vi "Convert64PinPGAToPattern.vi"(11 "64-Pin PGA":T3) -> (3 "Pattern":T1)   [LabVIEW 2012, in "Virtual-PGA.lvlib"]
uses:
  Virtual-PGA.lvlib
  Public/Controls/64PinPGAPattern.ctl
  Public/Controls/64PinPGAPads1-16.ctl
  Public/Controls/64PinPGAPad1-16.ctl
  Public/Controls/64PinPGAPads17-32.ctl
  Public/Controls/64PinPGAPad17-32.ctl
  Public/Controls/64PinPGAPads33-48.ctl
  Public/Controls/64PinPGAPad33-48.ctl
  Public/Controls/64PinPGAPads49-64.ctl
  Public/Controls/64PinPGAPad49-64.ctl
  Public/Controls/Pattern.ctl
  Public/Controls/Input.ctl
panel:
  # "Name:"
  # "Inputs:"
  # "Description:"
  # "Y4:"
  # "Y3:"
  # "Y2:"
  # "Y1:"
  # "49"
  # "50"
  # "51"
  # "52"
  # "53"
  # "54"
  # "55"
  # "56"
  # "57"
  # "58"
  # "59"
  # "60"
  # "61"
  # "62"
  # "63"
  # "64"
  # "1"
  # "2"
  # "3"
  # "4"
  # "5"
  # "6"
  # "7"
  # "8"
  # "9"
  # "10"
  # "11"
  # "12"
  # "13"
  # "14"
  # "15"
  # "16"
  # "32"
  # "31"
  # "30"
  # "29"
  # "28"
  # "27"
  # "26"
  # "25"
  # "24"
  # "23"
  # "22"
  # "21"
  # "20"
  # "19"
  # "18"
  # "17"
  # "48"
  # "47"
  # "46"
  # "45"
  # "44"
  # "43"
  # "42"
  # "41"
  # "40"
  # "39"
  # "38"
  # "37"
  # "36"
  # "35"
  # "34"
  # "33"
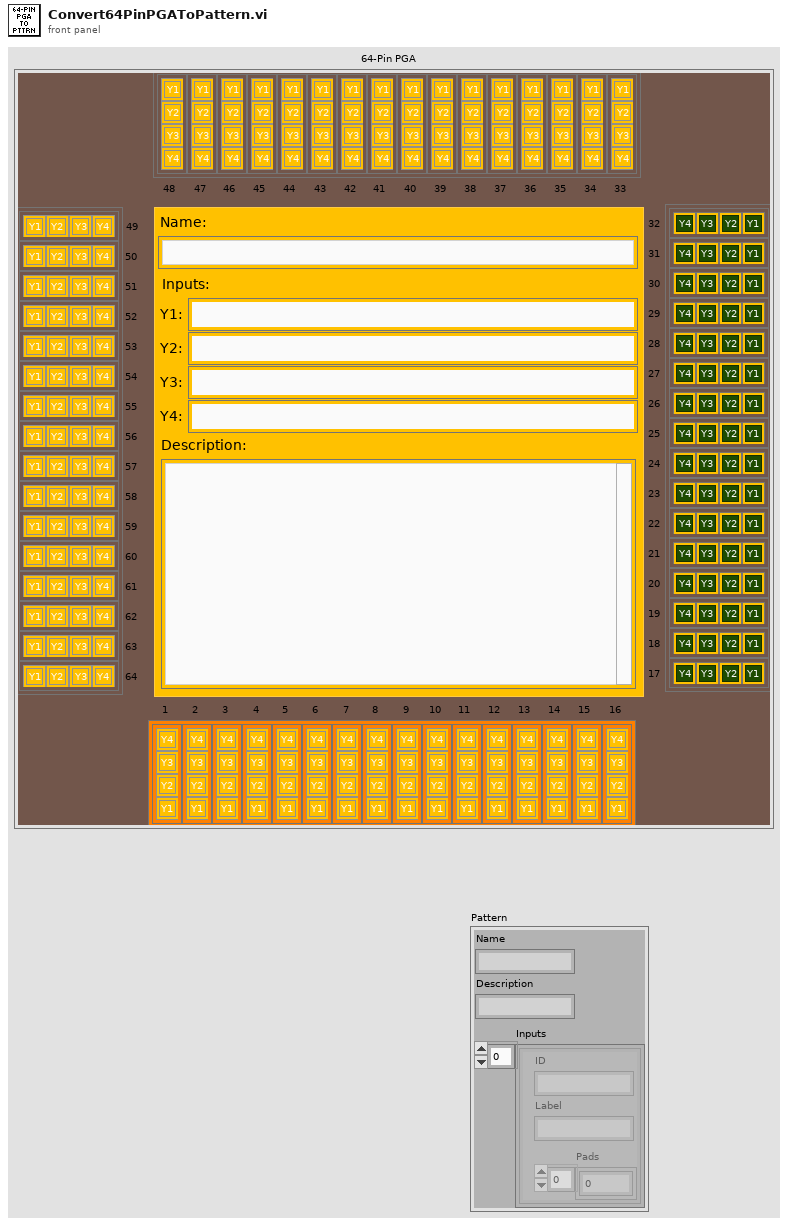
[diagram p1: front panel]
types:
  T1 = typedef "Virtual-PGA.lvlib/Pattern.ctl" = cluster{"Name":string, "Description":string, "Inputs":T2[]}
  T2 = typedef "Virtual-PGA.lvlib/Input.ctl" = cluster{"ID":string, "Label":string, "Pads":u32[]}
  T3 = typedef "Virtual-PGA.lvlib/64PinPGAPattern.ctl" = cluster{"Name":string, "Description":string, "Y1 Label":string, "Y2 Label":string, "Y3 Label":string, "Y4 Label":string, "Pads 1-16":T4, "Pads 17-32":T6, "Pads 33-48":T8, "Pads 49-64":T10}
  T4 = typedef "Virtual-PGA.lvlib/64PinPGAPads1-16.ctl" = T5[]
  T5 = typedef "Virtual-PGA.lvlib/64PinPGAPad1-16.ctl" = cluster{"Y1":bool, "Y2":bool, "Y3":bool, "Y4":bool}
  T6 = typedef "Virtual-PGA.lvlib/64PinPGAPads17-32.ctl" = T7[]
  T7 = typedef "Virtual-PGA.lvlib/64PinPGAPad17-32.ctl" = cluster{"Y1":bool, "Y2":bool, "Y3":bool, "Y4":bool}
  T8 = typedef "Virtual-PGA.lvlib/64PinPGAPads33-48.ctl" = T9[]
  T9 = typedef "Virtual-PGA.lvlib/64PinPGAPad33-48.ctl" = cluster{"Y1":bool, "Y2":bool, "Y3":bool, "Y4":bool}
  T10 = typedef "Virtual-PGA.lvlib/64PinPGAPads49-64.ctl" = T11[]
  T11 = typedef "Virtual-PGA.lvlib/64PinPGAPad49-64.ctl" = cluster{"Y1":bool, "Y2":bool, "Y3":bool, "Y4":bool}
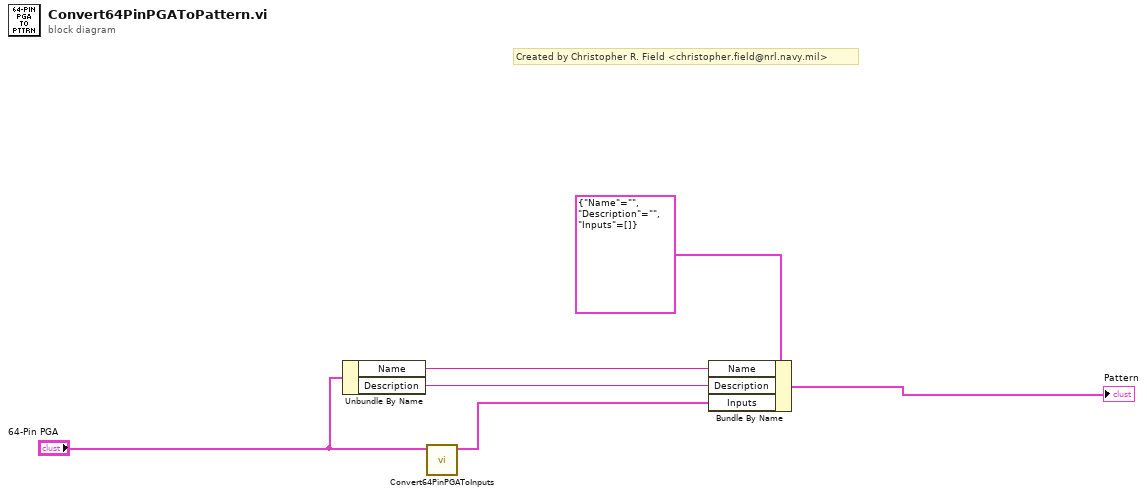
[diagram p0: block diagram]
diagram:
  # "Created by Christopher R. Field <christopher.field@nrl.navy.mil>"
  n1 = Unbundle By Name("64-Pin PGA") -> ("Name"=w3:string, "Description"=w2:string)
  n2 = call "Convert64PinPGAToInputs.vi"("64-Pin PGA"="64-Pin PGA") -> ("Inputs"=w1:T2[])  [unwired: 10 in]
  n3 = Bundle By Name(cluster=T1 {"Name"="", "Description"="", "Inputs"=[]} ("Pattern"), "Name"=w3, "Description"=w2, "Inputs"=w1) -> (→"Pattern":T1)
